vi "Write Input Level.vi"(8 "error in":errorcluster, 10 "Input Level":dbl, 11 "3300 in":refnum<class "3300.lvclass">) -> (0 "error out":errorcluster, 3 "3300 out":refnum<class "3300.lvclass">)   [LabVIEW 2019, in "3300.lvlib" / "3300.lvclass"]
uses:
  Library/3300.lvclass
  builds/Instruments/Electronic Load.lvlibp/Library/Electronic Load.lvclass
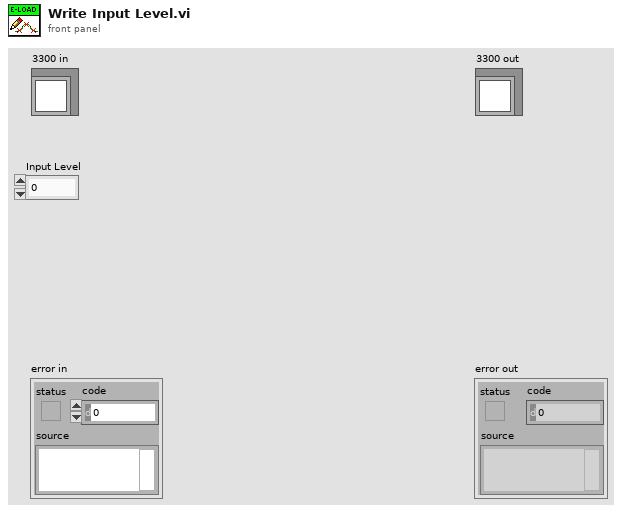
[diagram p1: front panel]
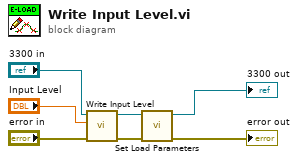
[diagram p0: block diagram]
diagram:
  n1 = call-parent "Write Input Level.vi"("error in"="error in", "Input Level"="Input Level", "Electronic Load in"="3300 in") -> ("error out"=w4:errorcluster, "Electronic Load out"=w3:refnum<class "3300.lvclass">)  [unwired: 7 in]
  n2 = call "Set Load Parameters.vi"("error in"=w4, "3300 in"=w3) -> ("error out"=→"error out":errorcluster, "3300 out"=→"3300 out":refnum<class "3300.lvclass">)  [unwired: 8 in]
